vi "DoProcess.vi"(8 "error in (no error)":errorcluster, 9 "MsgQ":refnum<queue>, 10 "AbstractionActor.lvclass":refnum<class "AbstractionActor.lvclass">, 11 "ActionC in":refnum<class "ActionC.lvclass">) -> (0 "error out":errorcluster, 2 "AbstractionActor.lvclass 2":refnum<class "AbstractionActor.lvclass">, 3 "ActionC out":refnum<class "ActionC.lvclass">)   [LabVIEW 2021, in "ActionC.lvclass"]
uses:
  ActionC.lvclass
  AbstractionActor/AbstractionActor.lvclass
  AbstractionMessage/AbstractionMessage.lvclass
  RealWorkActor/RealWorkActor.lvclass
  C:/Users/chrismadlax/Desktop/LVSampleCode/ActorModel/AbstractionActor/AbstractionActor.lvclass
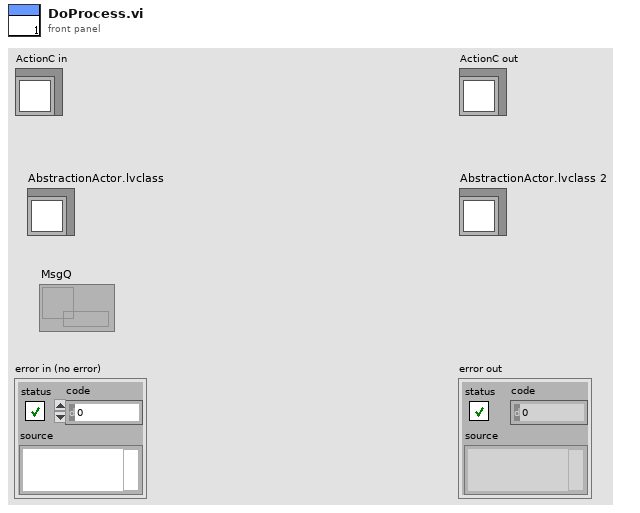
[diagram p1: front panel]
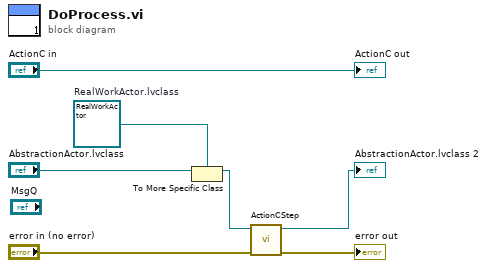
[diagram p0: block diagram]
diagram:
  w1 = refnum<class "RealWorkActor.lvclass"> refnum  # RealWorkActor.lvclass
  n1 = To More Specific Class(target class=w1, reference="AbstractionActor.lvclass") -> (specific class reference=w2:refnum<class "RealWorkActor.lvclass">)  [unwired: 1 in, 1 out]
  n2 = call "ActionCStep.vi"("error in (no error)"="error in (no error)", "RealWorkActor in"=w2) -> ("error out"=→"error out":errorcluster, "RealWorkActor out"=→"AbstractionActor.lvclass 2":refnum<class "RealWorkActor.lvclass">)  [unwired: 8 in]
  "ActionC out" <- "ActionC in"
